vi "OutputMixerMultiply.vi"(8 "Input Valid (T)":bool=TRUE, 10 "x":fxp<+/-,16,0>, 11 "y":i16) -> (3 "x*y":i16)   [LabVIEW 2013]
uses:
  <vilib>/rvi/FXPMathLib/FxpConvert/subVIs/nifxpmath_Convert_SimConfig.ctl
  <vilib>/fxp/LVFixedPointQuantizationPolicyTypeDef.ctl
  <vilib>/fxp/LVFixedPointOverflowPolicyTypeDef.ctl
  <vilib>/rvi/FXPMathLib/FxpConvert/simVIs/DllFxpConvertTemp_sub.vi
  <vilib>/rvi/FXPMathLib/FxpInterpret/XNode/nifxpmath_Interpret.xnode
  <vilib>/rvi/FXPMathLib/FxpConvert/XNode/nifxpmath_Convert.xnode
  <vilib>/rvi/FXPMathLib/FxpMul/XNode/nifxpmath_Multiplier.xnode
  <vilib>/rvi/FXPMathLib/sim/FxpSim.dll
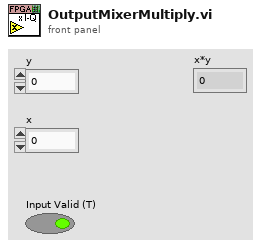
[diagram p1: front panel]
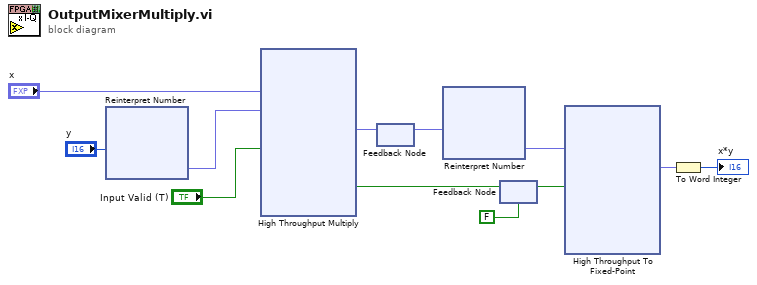
[diagram p0: block diagram]
diagram:
  n1 = xnode "Reinterpret Number"("x"="y") -> ("y"=w12:fxp<+/-,16,16>)
  n2 = xnode "High Throughput Multiply"("x"="x", "y"=w12, "input valid"="Input Valid (T)") -> ("x*y"=w3:fxp<+/-,32,16>, "output valid"=w8:bool)  [unwired: 1 in, 1 out]
  n3 = feedback #1() -> (w2:fxp<+/-,32,16>)  [unwired: 1 in]
  n4 = feedback-in #1(w3) -> ()
  n5 = xnode "Reinterpret Number"("x"=w2) -> ("y"=w1:fxp<+/-,32,20>)
  n6 = feedback #2(FALSE ("output valid")) -> (w7:bool)
  n7 = feedback-in #2(w8) -> ()
  n8 = xnode "High Throughput To Fixed-Point"("x"=w1, "input valid"=w7) -> ("y"=w10:fxp<+/-,16,16>)  [unwired: 1 in, 2 out]
  n9 = To Word Integer(number=w10) -> (16bit integer=→"x*y":i16)
